vi "Status Update.vi"() -> (3 "Status Cluster":T1)   [LabVIEW 2021]
uses:
  Controls/Pick & Place.ctl
  Global Variables/Index Status.vi
  Global Variables/TF Status.vi
  Global Variables/BF Status.vi
  Global Variables/Agitator Status.vi
  Global Variables/Insertion Status.vi
  Global Variables/Cutting Status.vi
  Global Variables/Pump Status.vi
  Global Variables/Measurement Status.vi
  Global Variables/Reject Status.vi
  Global Variables/RT GV.vi
  Global Variables/Pick & Place Status.vi
panel:
  out "Statuses":string[][](table)
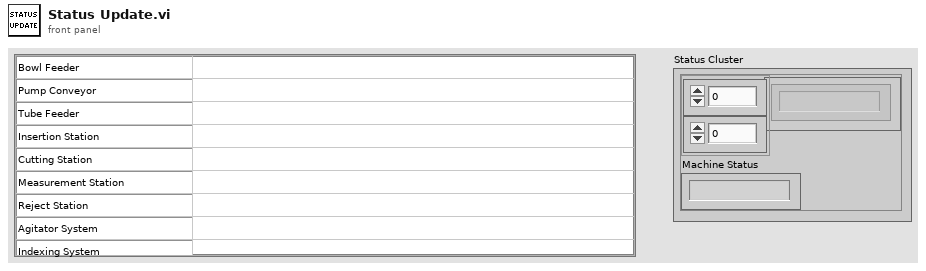
[diagram p1: front panel]
types:
  T1 = cluster{"Array":string[][], "Machine Status":string}
  T2 = typedef "Pick & Place.ctl" = enum16{"Initialise", "Singling ON", "Front Vertical SOL", "Rear Vertical SOL", "ON Rotary", "Front Vertical SOL_2", "Bowler ON", "Rear Vertical SOL_2", "OFF Rotary", "Done", "Error"}
  T3 = typedef "Bowl Feeder.ctl" = enum16{"Run", "Error"}
  T4 = typedef "Pump Feeder.ctl" = enum16{"Initialise", "Waiting For Pumps 1", "Gate Open", "Wait for Delay", "Gate Close", "Waiting For Pumps 2", "Done", "Error"}
  T5 = typedef "Tube Feeder.ctl" = enum16{"Initialise", "Gate Open", "Wait for Delay", "Gate Close", "Done", "Error"}
  T6 = typedef "Insertion.ctl" = enum16{"Initialise", "Clamp Fwd", "Clamp Delay", "CYL Fwd", "Wait for Delay", "CYL Rear", "Done", "Error"}
  T7 = typedef "Cutting v0.1.ctl" = enum16{"Initialise", "Clamp Fwd", "Clamp Delay", "Station Fwd", "Station Fwd Delay", "CYL Fwd", "Cut Delay", "CYL Rear", "Wait for Delay", "Station & Clamp Rear", "Done", "Error"}
  T8 = typedef "Measurement.ctl" = enum16{"Initialise", "CYL Fwd", "Wait for Delay", "CYL Rear", "Done", "Error"}
  T9 = typedef "Reject.ctl" = enum16{"Initialise", "CYL Fwd", "Wait for Delay", "CYL Rear", "Done", "Error"}
  T10 = typedef "Agitator.ctl" = enum16{"Initialise", "CYL Fwd", "Wait for Delay", "CYL Rear", "Wait For Rest", "Done", "Error"}
  T11 = typedef "Indexing.ctl" = enum16{"Initialise", "Go CCW", "Go CW (till stopper)", "Go CW (till complete)", "Return CCW", "Done", "Error"}
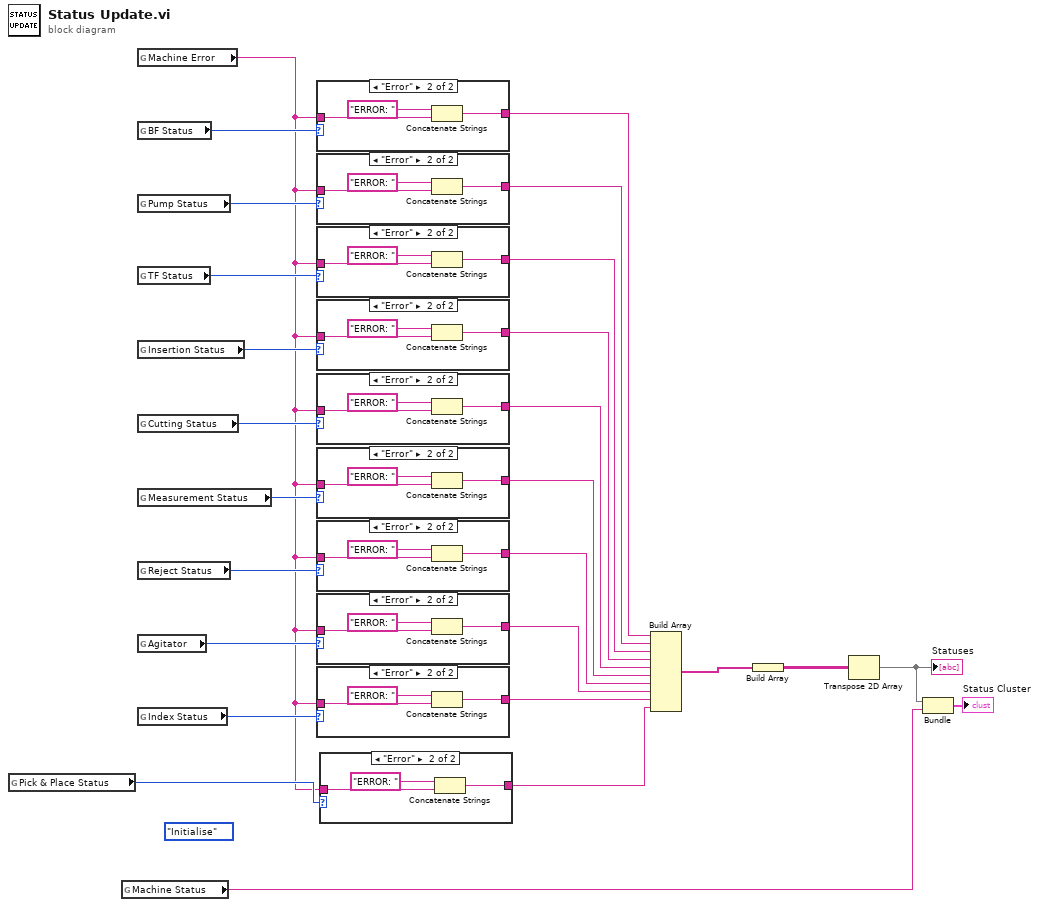
[diagram p0: block diagram]
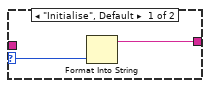
[diagram p2: hidden frame]
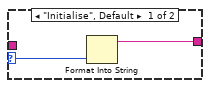
[diagram p3: hidden frame]
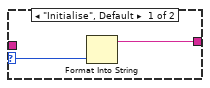
[diagram p4: hidden frame]
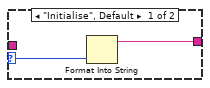
[diagram p5: hidden frame]
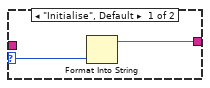
[diagram p6: hidden frame]
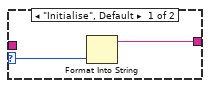
[diagram p7: hidden frame]
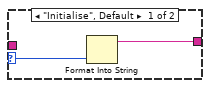
[diagram p8: hidden frame]
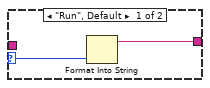
[diagram p9: hidden frame]
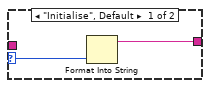
[diagram p10: hidden frame]
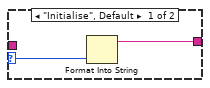
[diagram p11: hidden frame]
diagram:
  (unwired) Pick_&_Place."Initialise" ("Enum")
  n1 = global read "Pick & Place Status.vi" "Pick & Place Status"() -> (w2:T2)
  n2 = global read "RT GV.vi" "Machine Status"() -> (w5:string)
  n3 = global read "RT GV.vi" "Machine Error"() -> (w1:string)
  n4 = global read "BF Status.vi" "BF Status"() -> (w24:T3)
  n5 = global read "Pump Status.vi" "Pump Status"() -> (w19:T4)
  n6 = global read "TF Status.vi" "TF Status"() -> (w25:T5)
  n7 = global read "Insertion Status.vi" "Insertion Status"() -> (w22:T6)
  n8 = global read "Cutting Status.vi" "Cutting Status"() -> (w21:T7)
  n9 = global read "Measurement Status.vi" "Measurement Status"() -> (w20:T8)
  n10 = global read "Reject Status.vi" "Reject Status"() -> (w18:T9)
  n11 = global read "Agitator Status.vi" "Agitator"() -> (w23:T10)
  n12 = global read "Index Status.vi" "Index Status"() -> (w26:T11)
  n13 = case shown="\"Error\"" w24 {
    selector: w24 -> [w28 _]
    tunnel: [w27 w31] -> w17
    tunnel: w1 -> [_ w29]
    frame "Run", Default {
      n14 = Format Into String(w28) -> (resulting string=w27:string)  [unwired: 3 in, 1 out]
    }
    frame "Error" {
      n15 = Concatenate Strings("ERROR: " ("string"), w29) -> (w31:string)
    }
  }
  n16 = case shown="\"Error\"" w19 {
    selector: w19 -> [w33 _]
    tunnel: [w32 w35] -> w16
    tunnel: w1 -> [_ w34]
    frame "Initialise", Default {
      n17 = Format Into String(w33) -> (resulting string=w32:string)  [unwired: 3 in, 1 out]
    }
    frame "Error" {
      n18 = Concatenate Strings("ERROR: " ("string"), w34) -> (w35:string)
    }
  }
  n19 = case shown="\"Error\"" w25 {
    selector: w25 -> [w38 _]
    tunnel: [w37 w40] -> w15
    tunnel: w1 -> [_ w39]
    frame "Initialise", Default {
      n20 = Format Into String(w38) -> (resulting string=w37:string)  [unwired: 3 in, 1 out]
    }
    frame "Error" {
      n21 = Concatenate Strings("ERROR: " ("string"), w39) -> (w40:string)
    }
  }
  n22 = case shown="\"Error\"" w22 {
    selector: w22 -> [w43 _]
    tunnel: [w42 w45] -> w14
    tunnel: w1 -> [_ w44]
    frame "Initialise", Default {
      n23 = Format Into String(w43) -> (resulting string=w42:string)  [unwired: 3 in, 1 out]
    }
    frame "Error" {
      n24 = Concatenate Strings("ERROR: " ("string"), w44) -> (w45:string)
    }
  }
  n25 = case shown="\"Error\"" w21 {
    selector: w21 -> [w48 _]
    tunnel: [w47 w50] -> w13
    tunnel: w1 -> [_ w49]
    frame "Initialise", Default {
      n26 = Format Into String(w48) -> (resulting string=w47:string)  [unwired: 3 in, 1 out]
    }
    frame "Error" {
      n27 = Concatenate Strings("ERROR: " ("string"), w49) -> (w50:string)
    }
  }
  n28 = case shown="\"Error\"" w20 {
    selector: w20 -> [w53 _]
    tunnel: [w52 w55] -> w12
    tunnel: w1 -> [_ w54]
    frame "Initialise", Default {
      n29 = Format Into String(w53) -> (resulting string=w52:string)  [unwired: 3 in, 1 out]
    }
    frame "Error" {
      n30 = Concatenate Strings("ERROR: " ("string"), w54) -> (w55:string)
    }
  }
  n31 = case shown="\"Error\"" w18 {
    selector: w18 -> [w58 _]
    tunnel: [w57 w60] -> w11
    tunnel: w1 -> [_ w59]
    frame "Initialise", Default {
      n32 = Format Into String(w58) -> (resulting string=w57:string)  [unwired: 3 in, 1 out]
    }
    frame "Error" {
      n33 = Concatenate Strings("ERROR: " ("string"), w59) -> (w60:string)
    }
  }
  n34 = case shown="\"Error\"" w23 {
    selector: w23 -> [w63 _]
    tunnel: [w62 w65] -> w10
    tunnel: w1 -> [_ w64]
    frame "Initialise", Default {
      n35 = Format Into String(w63) -> (resulting string=w62:string)  [unwired: 3 in, 1 out]
    }
    frame "Error" {
      n36 = Concatenate Strings("ERROR: " ("string"), w64) -> (w65:string)
    }
  }
  n37 = case shown="\"Error\"" w26 {
    selector: w26 -> [w68 _]
    tunnel: [w67 w70] -> w9
    tunnel: w1 -> [_ w69]
    frame "Initialise", Default {
      n38 = Format Into String(w68) -> (resulting string=w67:string)  [unwired: 3 in, 1 out]
    }
    frame "Error" {
      n39 = Concatenate Strings("ERROR: " ("string"), w69) -> (w70:string)
    }
  }
  n40 = case shown="\"Error\"" w2 {
    selector: w2 -> [w73 _]
    tunnel: [w72 w75] -> w3
    tunnel: w1 -> [_ w74]
    frame "Initialise", Default {
      n41 = Format Into String(w73) -> (resulting string=w72:string)  [unwired: 3 in, 1 out]
    }
    frame "Error" {
      n42 = Concatenate Strings("ERROR: " ("string"), w74) -> (w75:string)
    }
  }
  n43 = Build Array(w17, w16, w15, w14, w13, w12, w11, w10, w9, w3) -> (w8:string[])
  n44 = Build Array(w8) -> (w7:string[][])
  n45 = Transpose 2D Array(2D array=w7) -> (transposed array=w6:string[][])
  "Statuses" <- w6
  n46 = Bundle(w6, "Machine Status"=w5) -> (→"Status Cluster":cluster{string[][], "Machine Status":string})  [unwired: 1 in]
